vi "RAW Image Buffer.vi"(7 "Actions":enum16{"Init", "Create", "Get", "Dispose"}(ring)=enum."Get", 8 "Error In":errorcluster) -> (0 "Error Out":errorcluster, 3 "Image Out":T1)   [LabVIEW 2018]
uses:
  <vilib>/vision/Image Controls.llb/IMAQ Image.ctl
  <resource>/objmgr/IMAQImage.rc
panel:
  out "Image Name":string
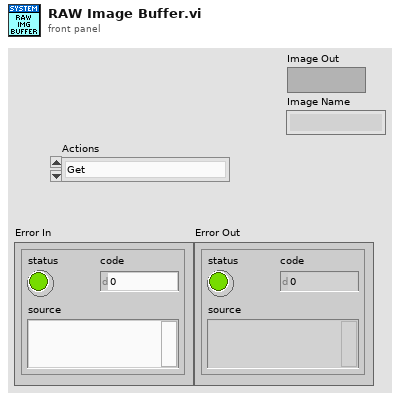
[diagram p1: front panel]
types:
  T1 = typedef "IMAQ Image.ctl" = refnum<image>
  T2 = typedef "Image Type" = u32
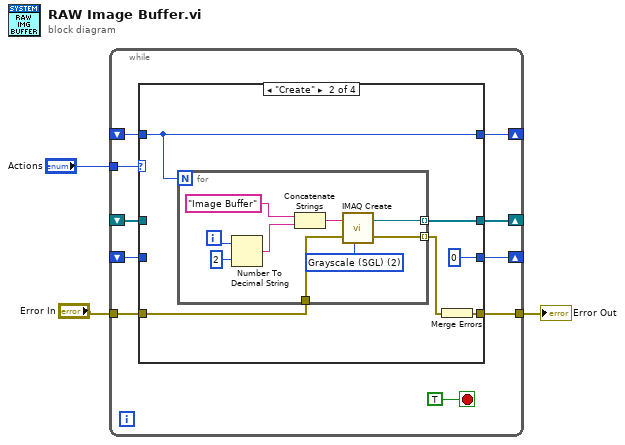
[diagram p0: block diagram]
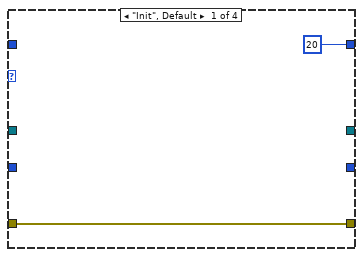
[diagram p2: hidden frame]
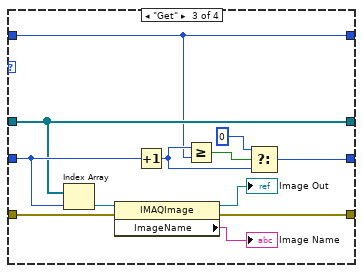
[diagram p3: hidden frame]
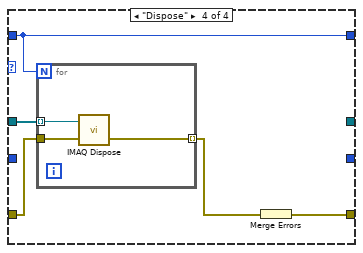
[diagram p4: hidden frame]
diagram:
  n1 = while {
    tunnel: "Actions" -> [w12]
    shift-right: [w11] -> _
    shift-left: _ -> [w10]
    shift-right: [w8] -> _
    shift-left: _ -> [w9]
    shift-right: [w7] -> _
    shift-left: _ -> [w6]
    tunnel: [w5] -> w2
    tunnel: "Error In" -> [w4]
    stop <- TRUE stop-if-true
    n2 = case shown="\"Create\"" w12 {
      tunnel: [_ w21 w41 _] -> w11
      tunnel: w10 -> [_ _ w41 w47]
      tunnel: w9 -> [_ _ w42 _]
      tunnel: [_ 0 w38 _] -> w8
      tunnel: [20 w19 w35 w46] -> w7
      tunnel: w6 -> [_ w19 w35 w46]
      tunnel: [w14 w17 w32 w43] -> w5
      tunnel: w4 -> [w14 w16 w31 w45]
      frame "Init", Default {
      }
      frame "Create" {
        n3 = for {
          N: w19 -> [_]
          tunnel: [w24] -> w21 mode=indexing
          tunnel: [w23] -> w18 mode=indexing
          tunnel: w16 -> [w22]
          i -> [w30]
          w28 = T2 2 items=["Grayscale (U8)", "Grayscale (I16)", "Grayscale (SGL)", "Complex (CSG)", "RGB (U32)", "HSL (U32)", "RGB (U64)", "Grayscale (U16)"] ("Image Type")
          n4 = Number To Decimal String(number=w30, width (-)=i16 2) -> (decimal integer string=w25:string)
          n5 = Concatenate Strings("Image Buffer" ("Image Name"), w25) -> (w26:string)
          n6 = call "IMAQ Create"("Image Name"=w26, "Image Type"=w28, "error in (no error)"=w22) -> ("New Image"=w24:T1, "error out"=w23:errorcluster)  [unwired: 2 in]
        }
        n7 = Merge Errors(w18) -> (w17:errorcluster)
      }
      frame "Get" {
        n8 = Index Array(array=w41, index=w42) -> (element=w40:T1)
        n9 = property class="IMAQImage"(reference=w40, error in=w31) -> (reference out=→"Image Out":T1, error out=w32:errorcluster, "ImageName"=→"Image Name":string)
        n10 = Increment(x=w42) -> (x+1=w36:i32)
        n11 = Greater Or Equal?(x=w36, y=w35) -> (x >= y?=w39:bool)
        n12 = Select(t=0, s=w39, f=w36) -> (s? t:f=w38:i32)
      }
      frame "Dispose" {
        n13 = for {
          N: w46 -> [_]
          tunnel: w47 -> [w50] mode=indexing
          tunnel: w45 -> [w49]
          tunnel: [w48] -> w44 mode=indexing
          n14 = call "IMAQ Dispose"("Image"=w50, "error in (no error)"=w49) -> ("error out"=w48:errorcluster)  [unwired: 4 in]
        }
        n15 = Merge Errors(w44) -> (w43:errorcluster)
      }
    }
  }
  "Error Out" <- w2
